vi "1ST_STAGE.vi"() -> (0 "Stage 1 Pressure":dbl(graph), 1 "Stage-I Temperature Transmitter (After Cooler)":dbl, 2 "Stage-I Pressure Transmitter":dbl, 3 "Stage 1 Temperature":dbl(graph), 4 "Stage 1 Coolant Temperature":dbl(graph), 5 "Stage-I Temperature Transmitter":dbl)   [LabVIEW 2014]
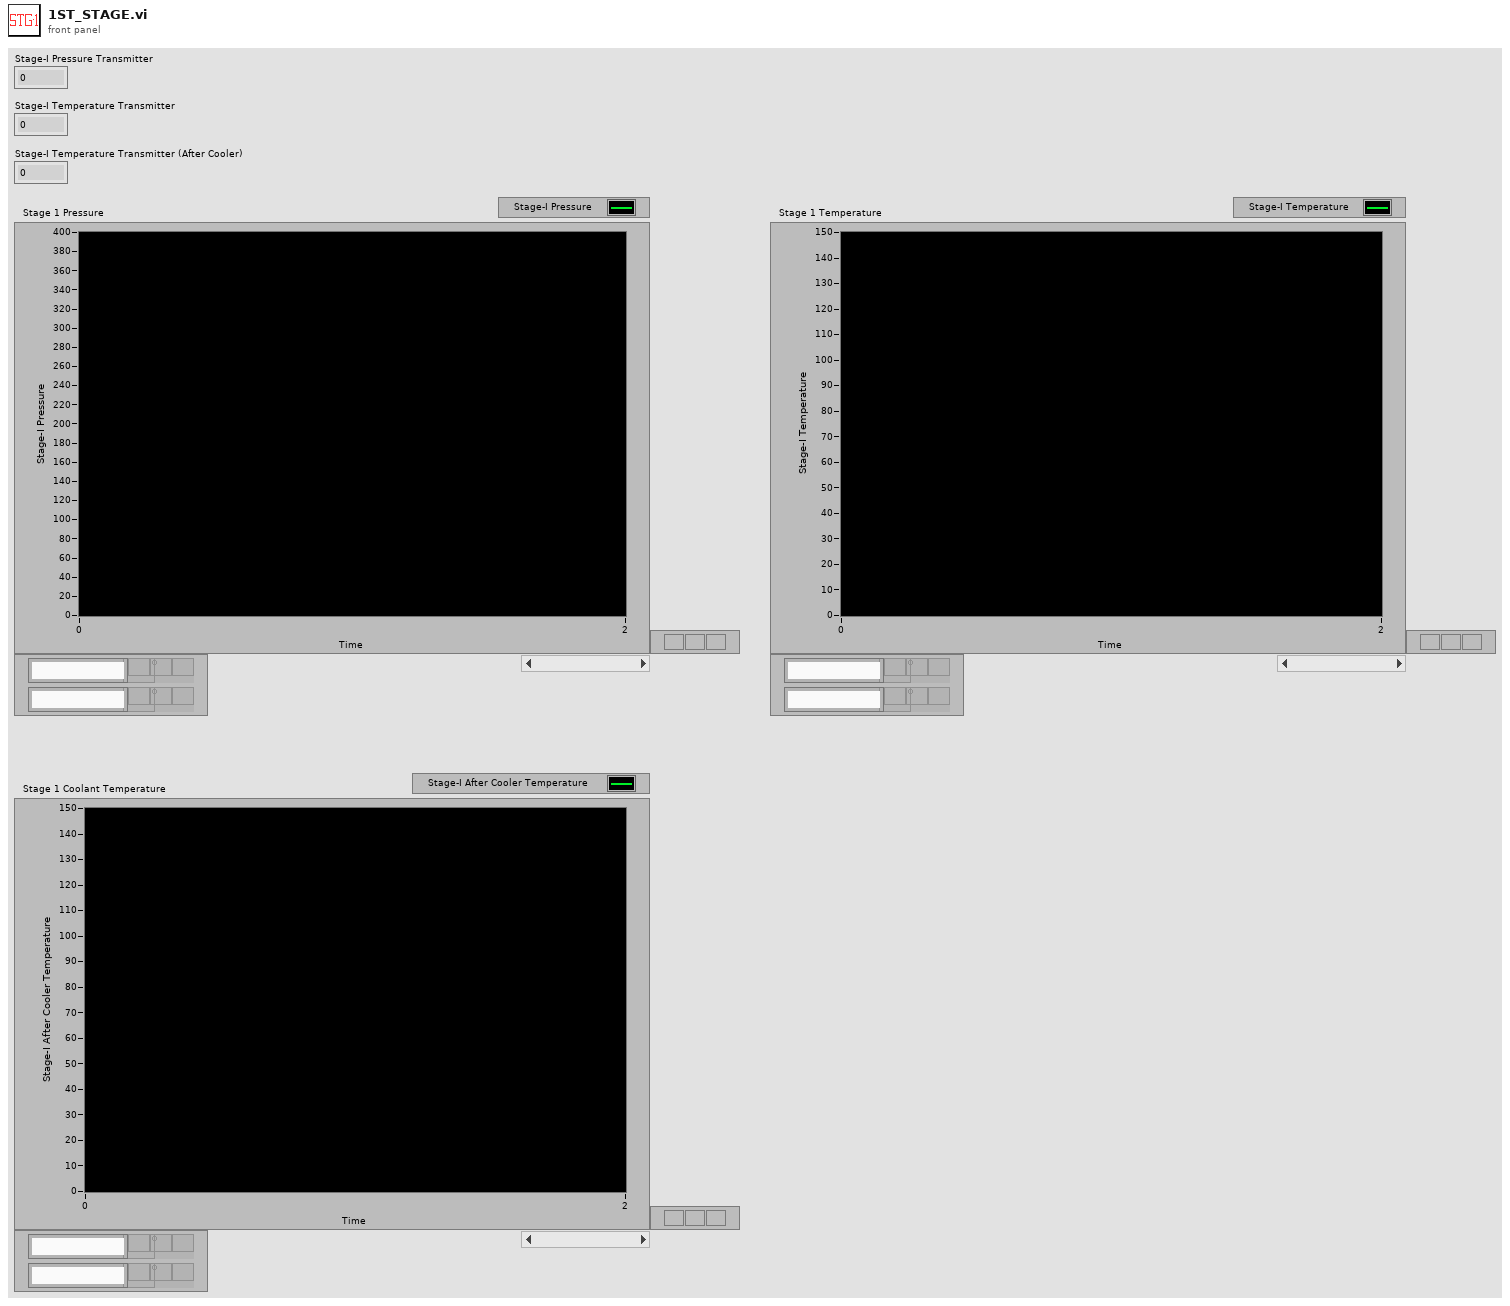
[diagram p1: front panel]
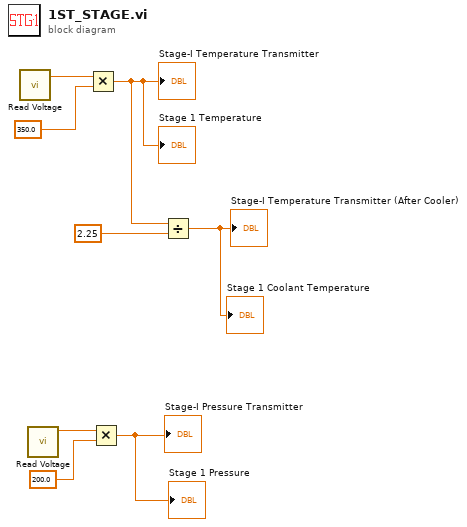
[diagram p0: block diagram]
diagram:
  n1 = call "Read Voltage.vi"() -> ("voltage"=w6:dbl)  [unwired: 6 in, 1 out]
  n2 = call "Read Voltage.vi"() -> ("voltage"=w8:dbl)  [unwired: 6 in, 1 out]
  n3 = Multiply(x=w6, y=350.0) -> (x*y=w2:dbl)
  "Stage-I Temperature Transmitter" <- w2
  "Stage 1 Temperature" <- w2
  n4 = Multiply(x=w8, y=200.0) -> (x*y=→"Stage-I Pressure Transmitter" →"Stage 1 Pressure":dbl)
  n5 = Divide(x=w2, y=2.25) -> (x/y=→"Stage-I Temperature Transmitter (After Cooler)" →"Stage 1 Coolant Temperature":dbl)
